vi "실습 2-3 수식노드.vi"() -> ()   [LabVIEW 2014]
panel:
  out "웨이브폼 그래프":dbl[](graph)
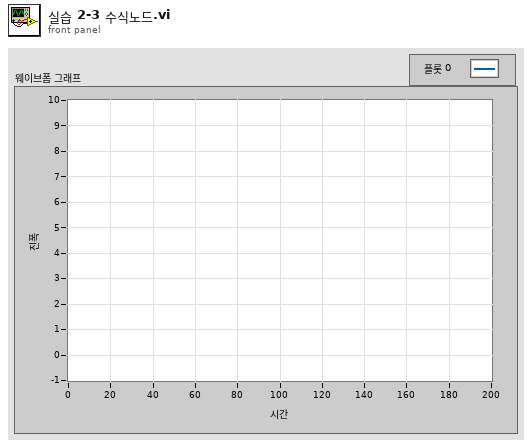
[diagram p1: front panel]
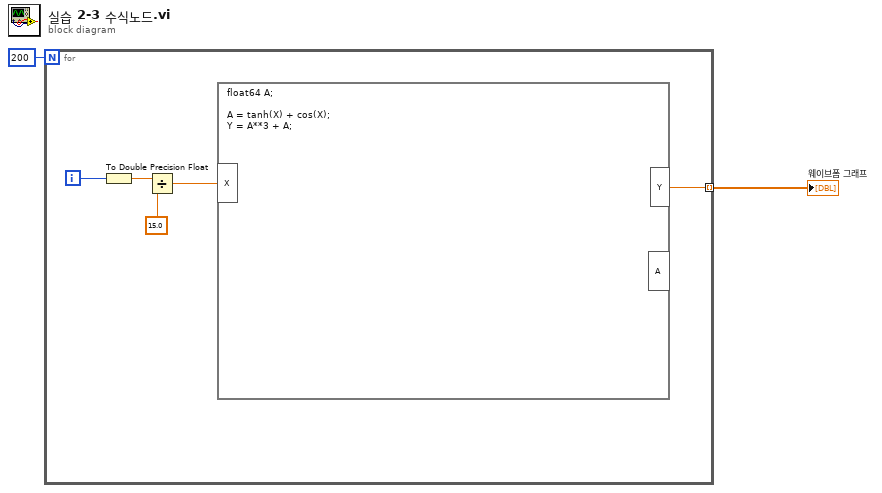
[diagram p0: block diagram]
diagram:
  n1 = for {
    N: 200 -> [_]
    tunnel: [w3] -> w1 mode=indexing
    i -> [w7]
    n2 = To Double Precision Float(number=w7) -> (double precision float=w6:dbl)
    n3 = Divide(x=w6, y=15.0) -> (x/y=w4:dbl)
    n4 = formula code="float64 A;\n\nA = tanh(X) + cos(X);\nY = A**3 + A;"("X"=w4) -> ("Y"=w3:dbl)  [unwired: 1 out]
  }
  "웨이브폼 그래프" <- w1
